vi "Write CAN FIFO.vi"(6 "FIFO Timestamps":T1, 8 "error in (no error)":errorcluster, 9 "Timeout (ms)":i32, 10 "Data":u8[](array[numeric]) format="%.0x", 11 "CIFTag in":refnum<class "CIF_NIChn_FifoCAN.lvclass">) -> (0 "error out":errorcluster, 1 "timed out?":bool, 3 "CIFTag out":refnum<class "CIF_NIChn_FifoCAN.lvclass">)   [LabVIEW 2021, in "CIF_NIChn_FifoCAN.lvclass"]
uses:
  CIF_NIChn_FifoCAN.lvclass
  NIChn/CIF_NIChn.lvclass
  <vilib>/CIF Foundation/CIF Channels/CIFChannels/CIFChannelCore.lvlib
  ChannelCommon/CIFFIFO/CIFfifo.lvclass
  D:/dev/Packages/Channel_Manager/src/CIF_NIChn/NIChn/CIF_NIChn.lvclass
  D:/dev/Packages/Channel_Manager/src/CIFChannels/CIFChannels.lvclass
  D:/dev/Packages/Channel_Manager/src/CIF_NIChn/FIFO_CAN/CIF_NIChn_FifoCAN.lvclass
  ChannelCommon/typedef/TimeStamps.ctl
  ChannelCommon/ChannelCommon.lvlib
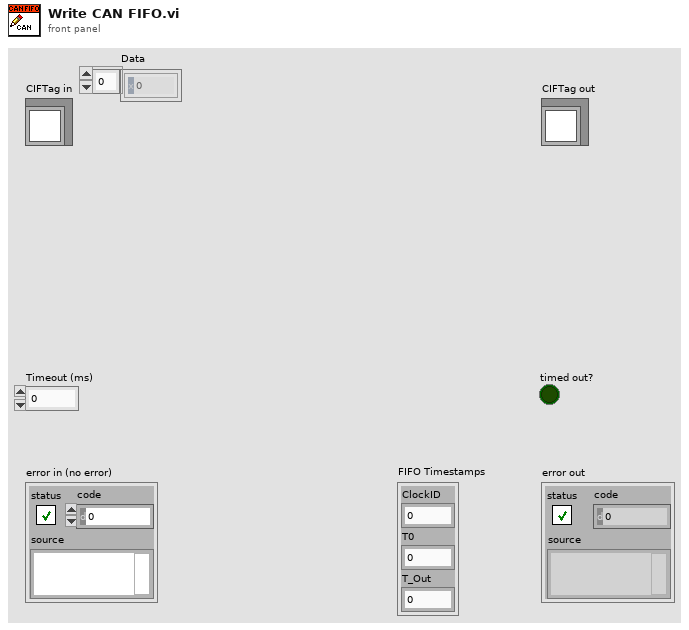
[diagram p1: front panel]
types:
  T1 = typedef "ChannelCommon.lvlib/TimeStamps.ctl" = cluster{"ClockID":u8, "T0":i64, "T_Out":i64}
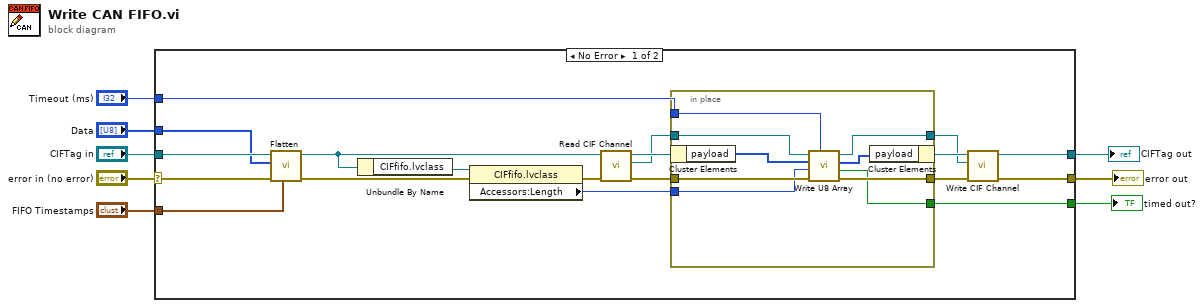
[diagram p0: block diagram]
diagram:
  n1 = case shown="No Error" "error in (no error)" {
    selector: "error in (no error)" -> [w12 w38]
    tunnel: [w18 w38] -> w7
    tunnel: [w23 w37] -> w5
    tunnel: "CIFTag in" -> [w15 w37]
    tunnel: [w27 _] -> w4
    tunnel: "Timeout (ms)" -> [w19 _]
    tunnel: "FIFO Timestamps" -> [w10 _]
    tunnel: "Data" -> [w9 _]
    frame No Error {
      n2 = call "Flatten.vi"("FIFO Timestamps"=w10, "error in (no error)"=w12, "Data in"=w9, "CIFTag in"=w15) -> ("error out"=w13:errorcluster, "CIFTag out"=w14:refnum<class "CIF_NIChn_FifoCAN.lvclass">)  [unwired: 6 in]
      n3 = Unbundle By Name(w14) -> ("CIFfifo.lvclass"=w17:refnum<class "CIFfifo.lvclass">)
      n4 = property class="CIFfifo.lvclass"(reference=w17, error in=w13) -> (error out=w16:errorcluster, "Accessors:Length"=w11:u64)  [unwired: 1 out]
      n5 = call "Read CIF Channel.vi"("error in (no error)"=w16, "CIFTag in"=w14) -> ("error out"=w25:errorcluster, "CIF Channel"=w21:refnum<k21>, "CIFTag out"=w26:refnum<class "CIF_NIChn_FifoCAN.lvclass">)  [unwired: 7 in]
      n6 = in-place {
        in-place-border: w25 -> [w36]
        in-place-border: [w35] -> w22
        in-place-border: [w34] -> w27
        in-place-border: w21 -> [w33]
        in-place-border: [w32] -> w20
        in-place-border: w19 -> [w31]
        in-place-border: w11 -> [w29]
        n7 = in-place-cluster #1(w26) -> ("payload"=w30:u8[])
        n8 = call <vilib>:"Write U8 Array.vi"("Timeout (ms)"=w31, "error in"=w36, "Number of Elements"=w29, "U8 Array in"=w30, "CIF Channel in"=w33) -> ("error out"=w35:errorcluster, "Timed out?"=w34:bool, "U8 Array out"=w28:u8[], "CIF Channel out"=w32:refnum<k21>)  [unwired: 3 in]
        n9 = in-place-cluster #1("payload"=w28) -> (w24:refnum<class "CIF_NIChn_FifoCAN.lvclass">)
      }
      n10 = call "Write CIF Channel.vi"("error in (no error)"=w22, "CIF Channel"=w20, "CIFTag in"=w24) -> ("error out"=w18:errorcluster, "CIFTag out"=w23:refnum<class "CIF_NIChn_FifoCAN.lvclass">)  [unwired: 7 in]
    }
    frame Error {
    }
  }
  "error out" <- w7
  "CIFTag out" <- w5
  "timed out?" <- w4
